vi "New Logger.vi"(7 "Logger Name":string, 8 "error in (no error)":errorcluster, 11 "Logger Output in":T1) -> (0 "error out":errorcluster)   [LabVIEW 2020, in "Global_logger.lvlib"]
uses:
  Global_logger.lvlib
  Logger Output.ctl
  Levels.ctl
  Level Meaning.ctl
  Sorting.ctl
  Logger Type.ctl
  Log Fields.ctl
  Event.ctl
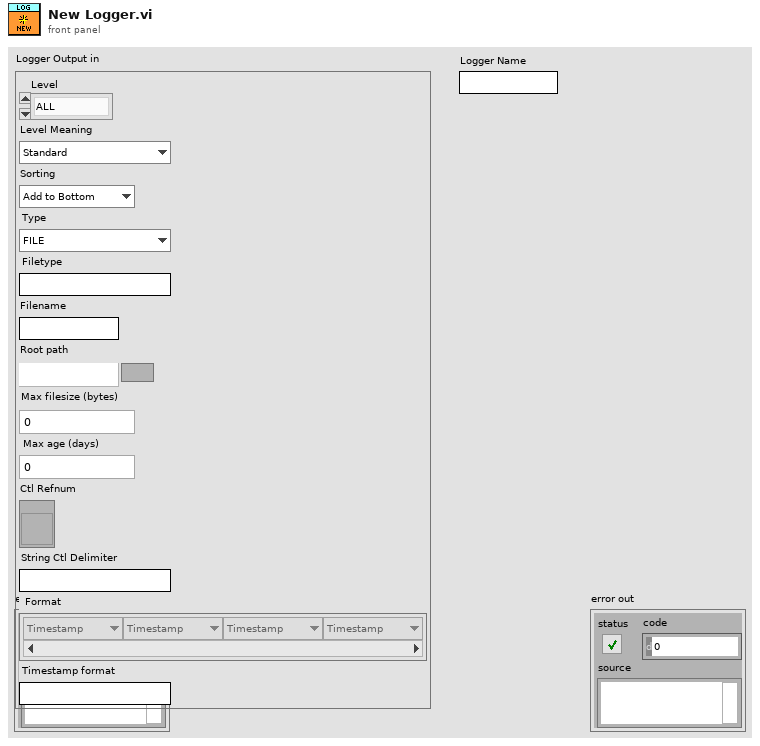
[diagram p1: front panel]
types:
  T1 = typedef "Global_logger.lvlib/Logger Output.ctl" = cluster{"Level":T2, "Level Meaning":T3, "Sorting":T4, "Type":T5, "Filetype":string, "Filename":string, "Root path":path, "Max filesize (bytes)":i32, "Max age (days)":i32, "Ctl Refnum":refnum<vi>, "String Ctl Delimiter":string, "Format":T6[], "Timestamp format":string}
  T2 = typedef "Global_logger.lvlib/Levels.ctl" = enum16{"ALL", "TRACE", "DEBUG", "INFO", "WARN", "ERROR", "FATAL", "OFF"}
  T3 = typedef "Global_logger.lvlib/Level Meaning.ctl" = enum16{"Standard", "Positive", "Exact"}
  T4 = typedef "Global_logger.lvlib/Sorting.ctl" = enum16{"Add to Bottom", "Add to Top"}
  T5 = typedef "Global_logger.lvlib/Logger Type.ctl" = enum16{"FILE", "UI"}
  T6 = typedef "Global_logger.lvlib/Log Fields.ctl" = enum16{"Timestamp", "Level", "Message", "Source VI", "Source App", "Logger Name"}
  T7 = typedef "Global_logger.lvlib/Event.ctl" = cluster{"Logger Name":string, "Time Stamp":timestamp, "Level":T2, "Source VI":string, "Message":string, "Source App":string}
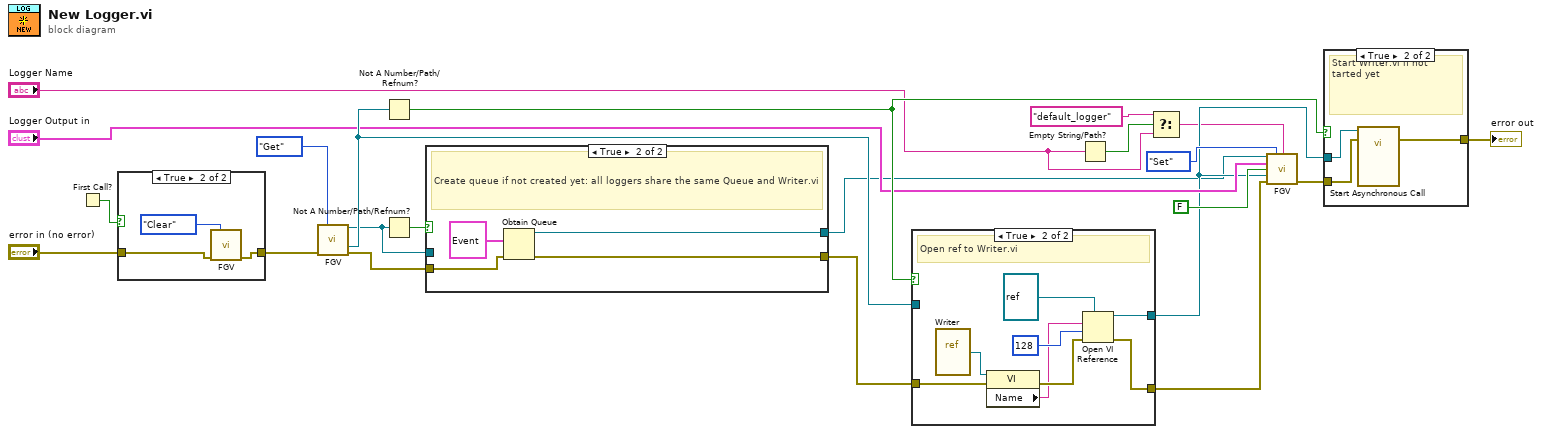
[diagram p0: block diagram]
diagram:
  n1 = First Call?() -> (First Call?: T/F=w3:bool)
  n2 = case shown="True" w3 {
    tunnel: "error in (no error)" -> [w23 w26]
    tunnel: [w23 w25] -> w1
    frame False {
    }
    frame True {
      n3 = call "FGV.vi"("Action"=enum16{"Get", "Set", "Clear"}."Clear", "error in (no error)"=w26) -> ("error out"=w25:errorcluster)  [unwired: 8 in, 5 out]
    }
  }
  n4 = call "FGV.vi"("Action"=enum16{"Get", "Set"}."Get", "error in (no error)"=w1) -> ("queue out"=w9:refnum<queue>, "Writer ref out"=w17:refnum<vi>, "error out"=w14:errorcluster)  [unwired: 8 in, 3 out]
  n5 = Not A Number/Path/Refnum?(number/path/refnum=w17) -> (NaN/Path/Refnum?=w16:bool)
  n6 = Not A Number/Path/Refnum?(number/path/refnum=w9) -> (NaN/Path/Refnum?=w18:bool)
  n7 = case shown="True" w18 {
    tunnel: [w28 w29] -> w8
    tunnel: w9 -> [w28 _]
    tunnel: w14 -> [w27 w31]
    tunnel: [w27 w30] -> w13
    frame False {
    }
    frame True {
      # "Create queue if not created yet: all loggers share the same Queue and Writer.vi"
      n8 = Obtain Queue(element data type=T7 {"Logger Name"="", "Time Stamp"=timestamp(0 s since 1904-01-01), "Level"=enum."ALL", "Source VI"="", "Message"="", "Source App"=""} ("Event"), error in (no error)=w31) -> (queue out=w29:refnum<queue>, error out=w30:errorcluster)  [unwired: 3 in, 1 out]
    }
  }
  n9 = case shown="True" w16 {
    tunnel: [w34 w37] -> w10
    tunnel: w17 -> [w34 _]
    tunnel: [w33 w36] -> w15
    tunnel: w13 -> [w33 w35]
    frame False {
    }
    frame True {
      # "Open ref to Writer.vi"
      n10 = vi-ref "Writer.vi"() -> (w38:refnum<vi>)
      n11 = property class="VI"(reference=w38, error in=w35) -> (error out=w41:errorcluster, "Name"=w39:string)  [unwired: 1 out]
      n12 = Open VI Reference(type specifier VI Refnum (for type only)=refnum<vi> refnum, vi path=w39, options=128, error in (no error)=w41) -> (vi reference=w37:refnum<vi>, error out=w36:errorcluster)  [unwired: 2 in]
    }
  }
  n13 = Empty String/Path?(string/path="Logger Name") -> (empty?=w7:bool)
  n14 = Select(t="default_logger", s=w7, f="Logger Name") -> (s? t:f=w6:string)
  n15 = call "FGV.vi"("queue in"=w8, "Action"=enum16{"Get", "Set"}."Set", "Logger Name"=w6, "Logger Output in"="Logger Output in", "Destroy Logger in"=FALSE, "Writer ref in"=w10, "error in (no error)"=w15) -> ("error out"=w20:errorcluster)  [unwired: 3 in, 5 out]
  n16 = case shown="True" w16 {
    tunnel: [w43 w46] -> w22
    tunnel: w20 -> [w43 w45]
    tunnel: w10 -> [_ w44]
    frame False {
    }
    frame True {
      # "Start Writer.vi if not tarted yet"
      n17 = call-by-ref "Start Asynchronous Call"(reference=w44, error in=w45) -> (error out=w46:errorcluster)  [unwired: 12 in, 1 out]
    }
  }
  "error out" <- w22
